vi "Experiment_2.vi"() -> ()   [LabVIEW 2019]
uses:
  <vilib>/measure/NI_MABase.lvlib
panel:
  in  "phase 3":dbl=90.0 format="%.2p"
  out "Received Wave 2":dynamicdata(graph)=[{"t0"=timestamp(0 s since 1904-01-01), "dt"=1e-05, "Y"=array[1000 elements], "attributes"=variant("NI_ChannelName"=variant(string "Filtered"))}]
  out "Received Wave 1":dynamicdata(graph)=[{"t0"=timestamp(0 s since 1904-01-01), "dt"=1e-05, "Y"=array[1000 elements], "attributes"=variant("NI_ChannelName"=variant(string "Filtered"))}]
  out "Added Modulated Wave":waveform(dbl)(graph)={"t0"=timestamp(0 s since 1904-01-01), "dt"=1e-05, "Y"=array[1000 elements]}
  out "Modulated Wave 2":waveform(dbl)(graph)={"t0"=timestamp(0 s since 1904-01-01), "dt"=1e-05, "Y"=array[1000 elements]}
  out "Modulated Wave 1":waveform(dbl)(graph)={"t0"=timestamp(0 s since 1904-01-01), "dt"=1e-05, "Y"=array[1000 elements]}
  in  "sampling info 4":cluster{"Fs":dbl, "#s":dbl}={"Fs"=100000.0, "#s"=1000.0} {"Fs" format="%.2p"}
  in  "sampling info 1":cluster{"Fs":dbl, "#s":dbl}={"Fs"=100000.0, "#s"=1000.0} {"Fs" format="%.2p"}
  in  "sampling info 3":cluster{"Fs":dbl, "#s":dbl}={"Fs"=100000.0, "#s"=1000.0} {"Fs" format="%.2p"}
  in  "sampling info 2":cluster{"Fs":dbl, "#s":dbl}={"Fs"=100000.0, "#s"=1000.0} {"Fs" format="%.2p"}
  in  "phase 2":dbl format="%.2p"
  in  "phase":dbl format="%.2p"
  out "Carrier Wave 2":waveform(dbl)(graph)={"t0"=timestamp(0 s since 1904-01-01), "dt"=1e-05, "Y"=array[1000 elements]}
  out "Modulating Wave 2":waveform(dbl)(graph)={"t0"=timestamp(0 s since 1904-01-01), "dt"=1e-05, "Y"=array[100000 elements]}
  out "Carrier Wave 1":waveform(dbl)(graph)={"t0"=timestamp(0 s since 1904-01-01), "dt"=1e-05, "Y"=array[1000 elements]}
  out "Modulating Wave 1":waveform(dbl)(graph)={"t0"=timestamp(0 s since 1904-01-01), "dt"=1e-05, "Y"=array[1000 elements]}
  in  "signal type 4":T1(ring)
  in  "amplitude 4":dbl=1.0 format="%0.2p"
  in  "frequency 4":dbl=10.0 format="%0.2p"
  in  "signal type 3":T1(ring)
  in  "amplitude 3":dbl=1.0 format="%0.2p"
  in  "frequency 3":dbl=10000.0 format="%0.2p"
  in  "signal type 2":T1(ring)
  in  "amplitude 2":dbl=1.0 format="%0.2p"
  in  "frequency 2":dbl=10000.0 format="%0.2p"
  in  "signal type":T1(ring)=enum."Triangle Wave"
  in  "amplitude":dbl=1.0 format="%0.2p"
  in  "frequency":dbl=10.0 format="%0.2p"
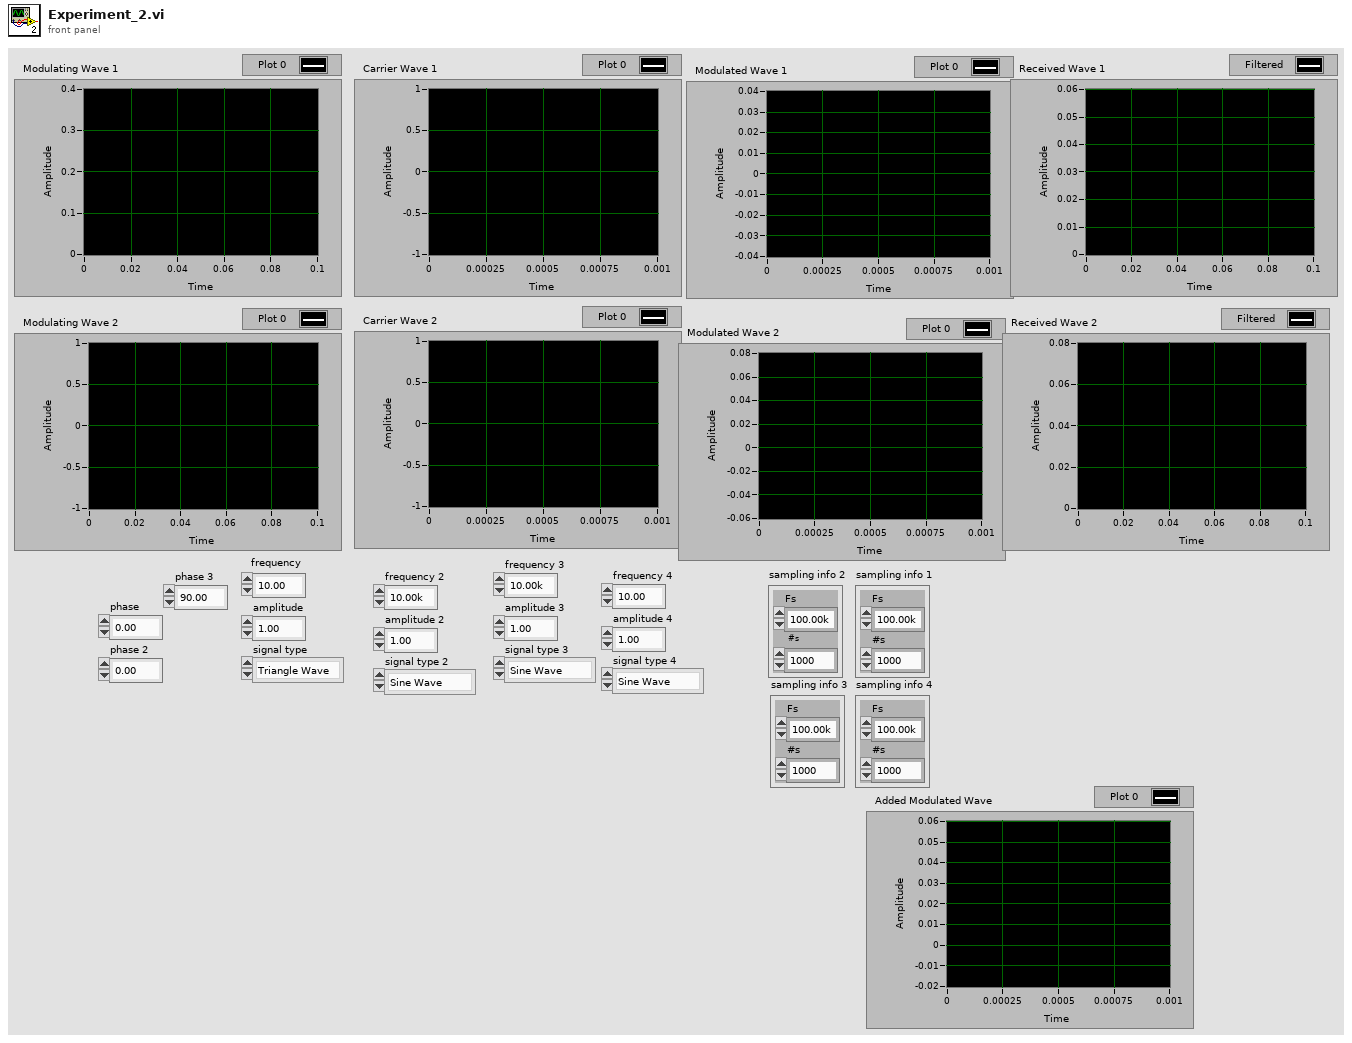
[diagram p1: front panel]
types:
  T1 = enum16{"Sine Wave", "Triangle Wave", "Square Wave", "Sawtooth Wave"}
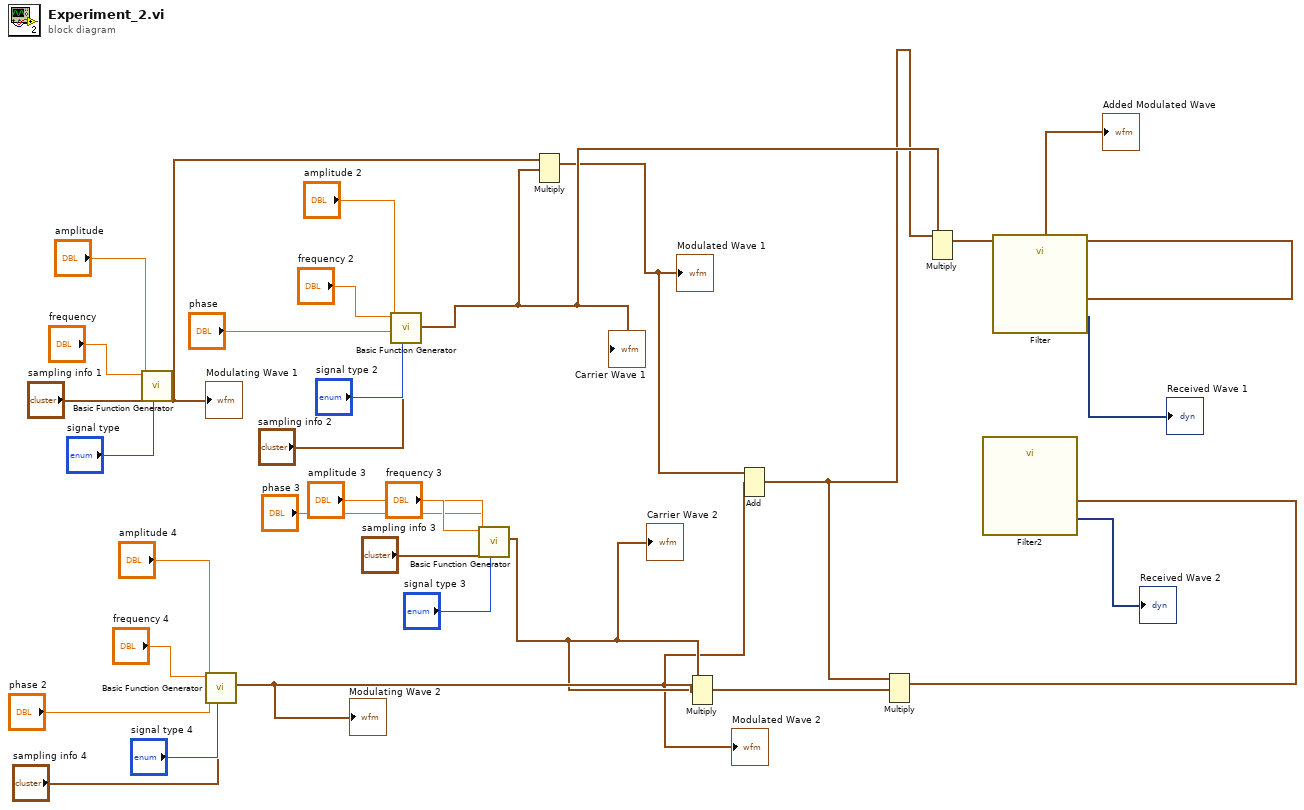
[diagram p0: block diagram]
diagram:
  n1 = call <vilib>:"Basic Function Generator.vi"("sampling info"="sampling info 1", "signal type"="signal type", "amplitude"="amplitude", "frequency"="frequency") -> ("signal out"=w16:waveform(dbl))  [unwired: 5 in, 2 out]
  "Modulating Wave 1" <- w16
  n2 = call <vilib>:"Basic Function Generator.vi"("sampling info"="sampling info 4", "signal type"="signal type 4", "phase"="phase 2", "amplitude"="amplitude 4", "frequency"="frequency 4") -> ("signal out"=w15:waveform(dbl))  [unwired: 4 in, 2 out]
  "Modulating Wave 2" <- w15
  n3 = call <vilib>:"Basic Function Generator.vi"("sampling info"="sampling info 2", "signal type"="signal type 2", "phase"="phase", "amplitude"="amplitude 2", "frequency"="frequency 2") -> ("signal out"=w10:waveform(dbl))  [unwired: 4 in, 2 out]
  "Carrier Wave 1" <- w10
  n4 = call <vilib>:"Basic Function Generator.vi"("sampling info"="sampling info 3", "signal type"="signal type 3", "phase"="phase 3", "amplitude"="amplitude 3", "frequency"="frequency 3") -> ("signal out"=w8:waveform(dbl))  [unwired: 4 in, 2 out]
  "Carrier Wave 2" <- w8
  n5 = Multiply(1:w10, 2:w16) -> (0:w6:waveform(dbl))  [unwired: 1 in, 1 out]
  "Modulated Wave 1" <- w6
  n6 = Multiply(1:w15, 2:w8) -> (0:w5:waveform(dbl))  [unwired: 1 in, 1 out]
  "Modulated Wave 2" <- w5
  n7 = Add(1:w5, 2:w6) -> (0:w9:waveform(dbl))  [unwired: 1 in, 1 out]
  n8 = Multiply(1:w8, 2:w9) -> (0:w7:waveform(dbl))  [unwired: 1 in, 1 out]
  n9 = Multiply(1:w10, 2:w9) -> (0:w4:waveform(dbl))  [unwired: 1 in, 1 out]
  "Added Modulated Wave" <- w4
  n10 = call "Filter2"("Signal"=w7) -> ("Filtered Signal"=→"Received Wave 2":dynamicdata)  [unwired: 9 in, 1 out]
  n11 = call "Filter"("Signal"=w4) -> ("Filtered Signal"=→"Received Wave 1":dynamicdata)  [unwired: 9 in, 1 out]
